vi "InterfaceManagement.vi"() -> ()   [LabVIEW 2019]
uses:
  02 Mode/SerialMode/SerialClass.lvclass
  02 Mode/TCPClientMode/TCPClientClass.lvclass
  02 Mode/TCPServerMode/TCPServerClass.lvclass
  29d042ba-0fcd-46a0-811e-070ad37dbe5e.vi
panel:
  out "新值":string
  in  "更新显示？":bool
  in  "停止":bool
  in  "连接显示":string(tree)
  # "针对客服端/服务端\n不能检测是否可用\n客服端连接服务端的情况，当前无法联动删除"
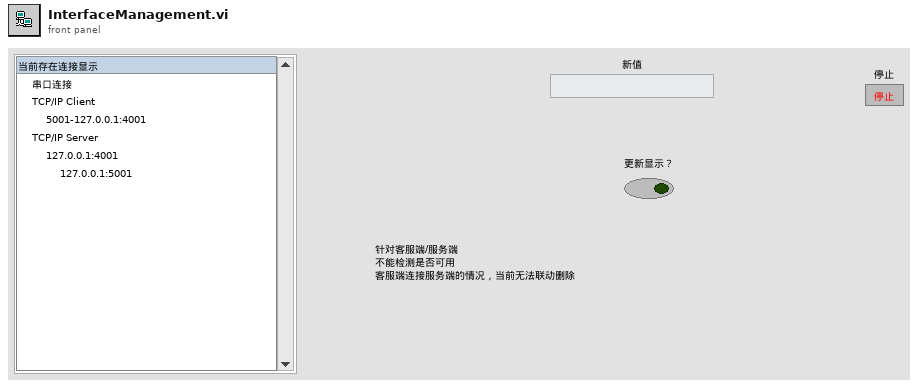
[diagram p1: front panel]
types:
  T1 = typedef "队列枚举1.ctl" = enum16{"接口管理页队列", "服务侦听页队列", "主页队列"}
  T2 = typedef "队列枚举.ctl" = enum16{"ini", "读", "写"}
  T3 = typedef "串口枚举.ctl" = enum16{"ini", "增", "删", "查", "改"}
  T4 = cluster{"串口名":string, "串口类":refnum<class "SerialClass.lvclass">}
  T5 = cluster{"客服名":string, "客服类":refnum<class "TCPClientClass.lvclass">}
  T6 = cluster{"服务名":string, "服务类":refnum<class "TCPServerClass.lvclass">}
  T7 = cluster{"识别名称":string, "记录":cluster{"通讯状态":bool, "记录上限":dbl, "报文记录":string[]}}
  T8 = enum16{"ini", "增", "删", "查", "改-通讯状态", "改-记录上限", "增-报文", "清空报文记录", "清空全部记录"}
  T9 = map{string, refnum<class "TCPClientClass.lvclass">}
  T10 = map{string, refnum<class "TCPServerClass.lvclass">}
  T11 = cluster{"未找到?":bool, "服务类":refnum<class "TCPServerClass.lvclass">}
  T12 = cluster{"字符串":string, "TCPServerClass输出":refnum<class "TCPServerClass.lvclass">}
  T13 = typedef "LVPoint32TypeDef.ctl" = cluster{"Horizontal":i32, "Vertical":i32}
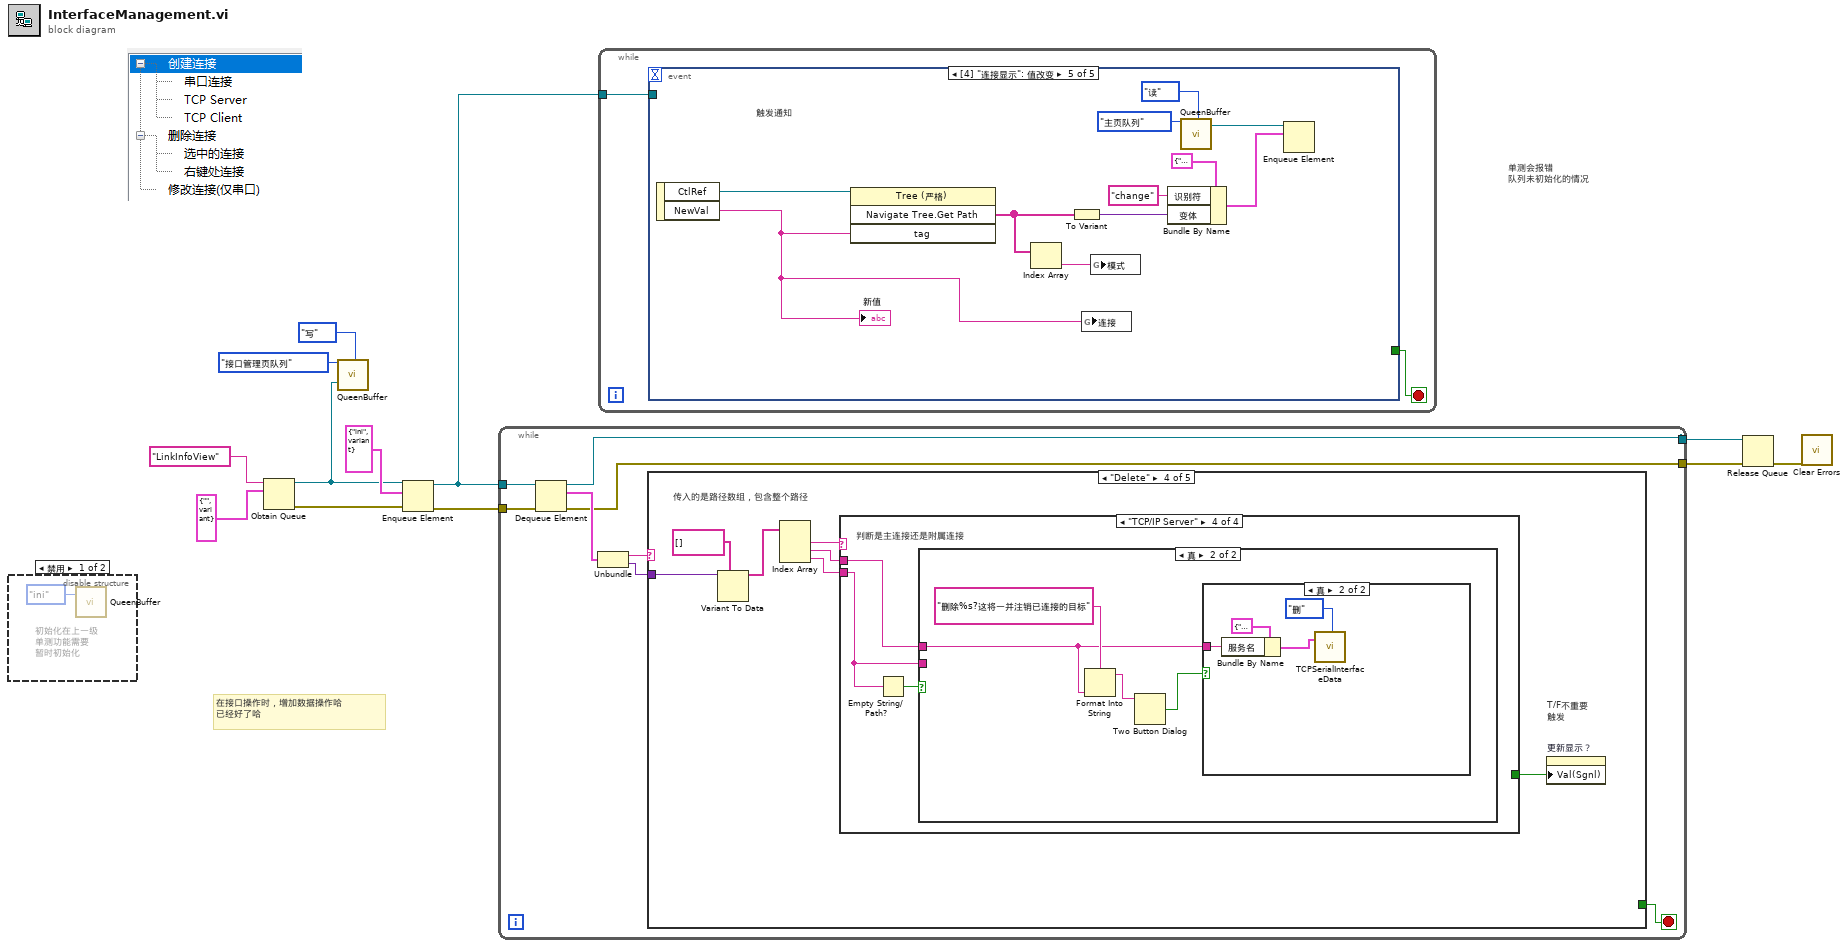
[diagram p0: block diagram]
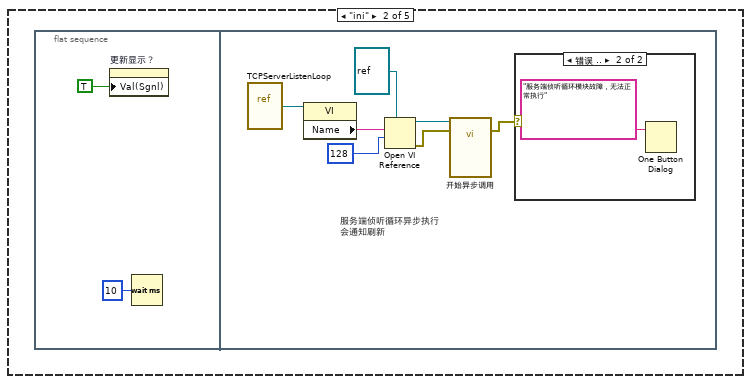
[diagram p4: hidden frame]
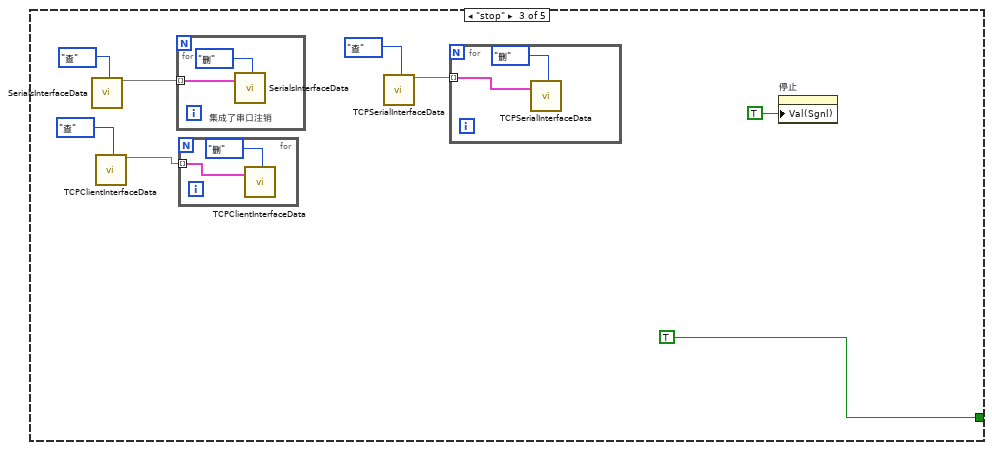
[diagram p6: hidden frame]
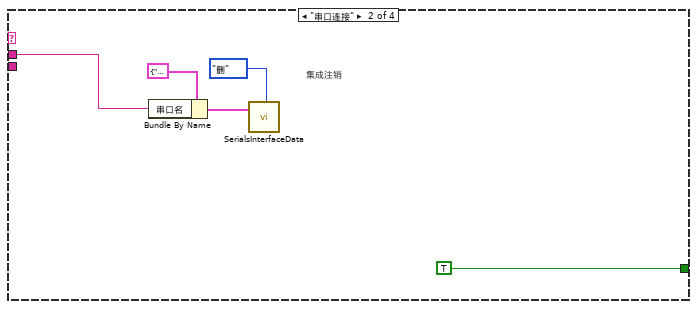
[diagram p8: hidden frame]
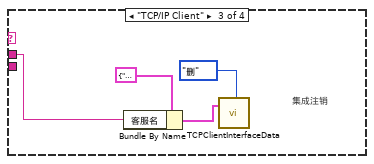
[diagram p9: hidden frame]
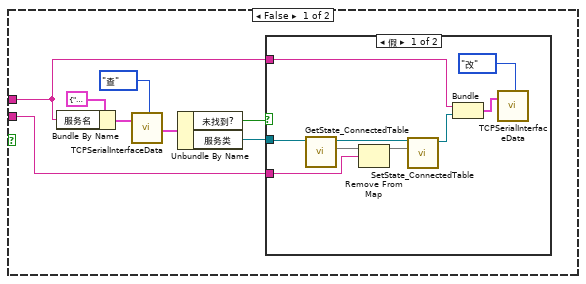
[diagram p10: hidden frame]
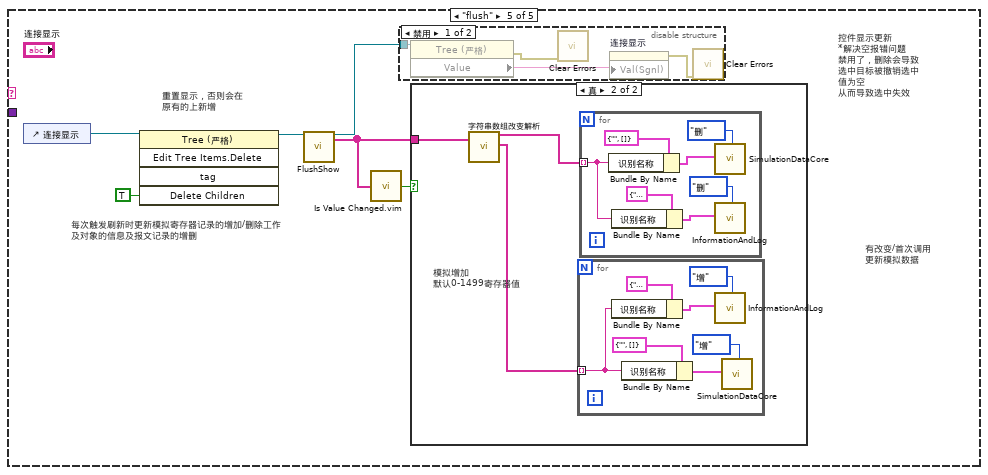
[diagram p13: hidden frame]
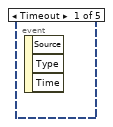
[diagram p16: hidden frame]
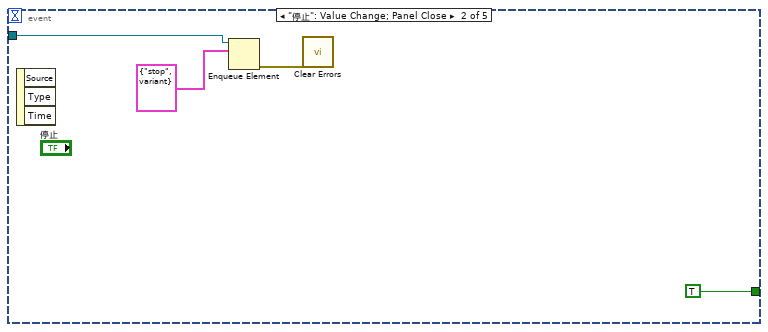
[diagram p17: hidden frame]
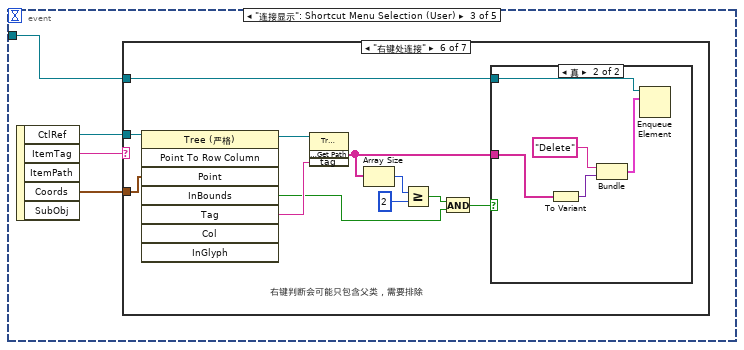
[diagram p18: hidden frame]
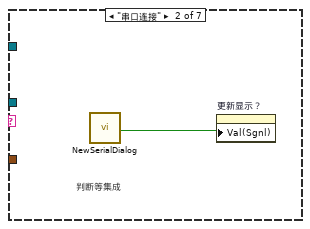
[diagram p20: hidden frame]
diagram:
  # "单测会报错\n队列未初始化的情况"
  # "在接口操作时，增加数据操作哈\n已经好了哈"
  n1 = disable-structure shown="禁用" {
    frame Disabled {
      # "初始化在上一级\n单测功能需要\n暂时初始化"
      n2 = call "QueenBuffer.vi"(1:队列枚举."ini" ("队列枚举")) -> ()  [unwired: 18 in, 1 out]
    }
    frame Enabled {
    }
  }
  n3 = Obtain Queue(name (unnamed)="LinkInfoView" ("名称（未命名）"), element data type=cluster{string, variant} {"", variant}) -> (queue out=w2:refnum<queue>, error out=w11:errorcluster)  [unwired: 3 in, 1 out]
  n4 = call "QueenBuffer.vi"("名称"=队列枚举1."接口管理页队列", "目标队列输入"=w2, "操作"=队列枚举."写") -> ()  [unwired: 16 in, 1 out]
  n5 = Enqueue Element(queue=w2, element=cluster{string, variant} {"ini", variant} ("元素"), error in (no error)=w11) -> (queue out=w10:refnum<queue>, error out=w9:errorcluster)  [unwired: 1 in, 1 out]
  n6 = while {
    tunnel: w10 -> [w21]
    tunnel: w9 -> [w20]
    tunnel: [w16] -> w8
    tunnel: [w15] -> w7
    stop <- w14 stop-if-true
    n7 = Dequeue Element(queue=w21, error in (no error)=w20) -> (queue out=w16:refnum<queue>, element=w19:cluster{string, variant}, error out=w15:errorcluster)  [unwired: 1 in, 1 out]
    n8 = Unbundle(w19) -> (w18:string, w17:variant)
    n9 = case shown="\"Delete\"" w18 {
      tunnel: w17 -> [_ _ _ w52 _]
      tunnel: [_ _ TRUE ("停止") _ _] -> w14
      frame Default {
      }
      frame "ini" {
        n10 = flat-sequence {
          frame #0 {
            n11 = property on="更新显示？" class="Bool (严格)"("Val(Sgnl)"=TRUE ("更新显示？")) -> ()  [unwired: 2 in, 2 out]
            n12 = Wait (ms)(milliseconds to wait=u32 10 ("等待时间（毫秒）")) -> ()  [unwired: 1 out]
          }
          frame #1 {
            # "服务端侦听循环异步执行\n会通知刷新"
            n13 = vi-ref "TCPServerListenLoop.vi"() -> (w30:refnum<vi>)
            n14 = property class="VI"(reference=w30) -> ("Name"=w29:string)  [unwired: 1 in, 2 out]
            n15 = Open VI Reference(type specifier VI Refnum (for type only)=refnum<vi> refnum ("类型说明符VI引用句柄（仅用于类型）"), vi path=w29, options=128 ("选项")) -> (vi reference=w28:refnum<vi>, error out=w27:errorcluster)  [unwired: 3 in]
            n16 = call-by-ref "开始异步调用"(reference=w28, error in=w27) -> (error out=w24:errorcluster)  [unwired: 20 in, 1 out]
            n17 = case shown="错误 .." w24 {
              frame No Error {
              }
              frame Error {
                n18 = One Button Dialog(message="服务端侦听循环模块故障，无法正常执行" ("消息")) -> ()  [unwired: 1 in, 1 out]
              }
            }
          }
        }
      }
      frame "stop" {
        n19 = call "SerialsInterfaceData.vi"("串口枚举"=串口枚举."查") -> ("串口表"=w37:map{string, refnum<class "SerialClass.lvclass">})  [unwired: 17 in, 1 out]
        n20 = call "TCPClientInterfaceData.vi"("客服接口枚举"=enum16{"ini", "增", "删", "查", "改"}."查") -> ("客服表"=w34:T9)  [unwired: 17 in, 1 out]
        n21 = for {
          tunnel: w37 -> [w44] mode=indexing
          # "集成了串口注销"
          n22 = call "SerialsInterfaceData.vi"("信息"=w44, "串口枚举"=串口枚举."删") -> ()  [unwired: 16 in, 2 out]
        }
        n23 = for {
          tunnel: w34 -> [w42] mode=indexing
          n24 = call "TCPClientInterfaceData.vi"("信息"=w42, "客服接口枚举"=enum16{"ini", "增", "删", "查", "改"}."删") -> ()  [unwired: 16 in, 2 out]
        }
        n25 = call "TCPSerialInterfaceData.vi"("客服接口枚举"=enum16{"ini", "增", "删", "查", "改", "腾笼换鸟"}."查") -> ("服务表"=w33:T10)  [unwired: 17 in, 1 out]
        n26 = for {
          tunnel: w33 -> [w40] mode=indexing
          n27 = call "TCPSerialInterfaceData.vi"("信息"=w40, "客服接口枚举"=enum16{"ini", "增", "删", "查", "改", "腾笼换鸟"}."删") -> ()  [unwired: 16 in, 2 out]
        }
        n28 = property on="停止" class="Bool (严格)"("Val(Sgnl)"=TRUE ("值(信号)")) -> ()  [unwired: 2 in, 2 out]
      }
      frame "Delete" {
        # "T/F不重要\n触发"
        # "传入的是路径数组，包含整个路径"
        n29 = Variant To Data(type=string[] [], Variant=w52) -> (data=w50:string[])  [unwired: 1 in, 1 out]
        n30 = Index Array(array=w50) -> (element #1=w49:string, element #2=w48:string, element #3=w47:string)  [unwired: 3 in]
        n31 = case shown="\"TCP/IP Server\"" w49 {
          tunnel: w48 -> [_ w55 w59 w63]
          tunnel: w47 -> [_ _ _ w62]
          tunnel: [_ TRUE _ _] -> w46
          frame Default {
          }
          frame "串口连接" {
            # "集成注销"
            n32 = Bundle By Name(cluster=T4 {"串口名"="", "串口类"=refnum} ("信息"), "串口名"=w55) -> (w54:T4)
            n33 = call "SerialsInterfaceData.vi"("信息"=w54, "串口枚举"=串口枚举."删") -> ()  [unwired: 16 in, 2 out]
          }
          frame "TCP/IP Client" {
            # "集成注销"
            n34 = Bundle By Name(cluster=T5 {"客服名"="", "客服类"=refnum} ("信息"), "客服名"=w59) -> (w58:T5)
            n35 = call "TCPClientInterfaceData.vi"("信息"=w58, "客服接口枚举"=enum16{"ini", "增", "删", "查", "改"}."删") -> ()  [unwired: 16 in, 2 out]
          }
          frame "TCP/IP Server" {
            # "判断是主连接还是附属连接"
            n36 = Empty String/Path?(string/path=w62) -> (empty?=w64:bool)
            n37 = case shown="真" w64 {
              tunnel: w63 -> [w66 w83]
              tunnel: w62 -> [w65 _]
              frame False {
                n38 = Bundle By Name(cluster=T6 {"服务名"="", "服务类"=refnum} ("信息"), "服务名"=w66) -> (w70:T6)
                n39 = call "TCPSerialInterfaceData.vi"("信息"=w70, "客服接口枚举"=enum16{"ini", "增", "删", "查", "改", "腾笼换鸟"}."查") -> ("查找结果"=w69:T11)  [unwired: 16 in, 1 out]
                n40 = Unbundle By Name(w69) -> ("未找到?"=w68:bool, "服务类"=w67:refnum<class "TCPServerClass.lvclass">)
                n41 = case shown="假" w68 {
                  tunnel: w67 -> [w81 _]
                  tunnel: w66 -> [w74 _]
                  tunnel: w65 -> [w78 _]
                  frame False {
                    n42 = call-dynamic "GetState_ConnectedTable.vi"("TCPServerClass输入"=w81) -> ("连接端ID表"=w79:map{string, refnum<k5>}, "TCPServerClass输出"=w80:refnum<class "TCPServerClass.lvclass">)  [unwired: 8 in, 1 out]
                    n43 = Remove From Map(10:w78, 11:w79) -> (3:w77:map{string, refnum<k5>})  [unwired: 2 out]
                    n44 = call-dynamic "SetState_ConnectedTable.vi"("连接端ID表"=w77, "TCPServerClass输入"=w80) -> ("TCPServerClass输出"=w75:refnum<class "TCPServerClass.lvclass">)  [unwired: 8 in, 1 out]
                    n45 = Bundle("字符串"=w74, "TCPServerClass输出"=w75) -> (w73:T12)  [unwired: 1 in]
                    n46 = call "TCPSerialInterfaceData.vi"("信息"=w73, "客服接口枚举"=enum16{"ini", "增", "删", "查", "改", "腾笼换鸟"}."改") -> ()  [unwired: 16 in, 2 out]
                  }
                  frame True {
                  }
                }
              }
              frame True {
                n47 = Format Into String(format string="删除%s?这将一并注销已连接的目标" ("消息"), w83) -> (resulting string=w82:string)  [unwired: 2 in, 1 out]
                n48 = Two Button Dialog(message=w82) -> (T button?=w85:bool)  [unwired: 2 in]
                n49 = case shown="真" w85 {
                  tunnel: w83 -> [_ w87]
                  frame False {
                  }
                  frame True {
                    n50 = Bundle By Name(cluster=T6 {"服务名"="", "服务类"=refnum} ("信息"), "服务名"=w87) -> (w86:T6)
                    n51 = call "TCPSerialInterfaceData.vi"("信息"=w86, "客服接口枚举"=enum16{"ini", "增", "删", "查", "改", "腾笼换鸟"}."删") -> ()  [unwired: 16 in, 2 out]
                  }
                }
              }
            }
          }
        }
        n52 = property on="更新显示？" class="Bool (严格)"("Val(Sgnl)"=w46) -> ()  [unwired: 2 in, 2 out]
      }
      frame "flush" {
        # "每次触发刷新时更新模拟寄存器记录的增加/删除工作\n及对象的信息及报文记录的增删"
        # "有改变/首次调用\n更新模拟数据"
        # "重置显示，否则会在\n原有的上新增"
        # "控件显示更新\n*解决空报错问题\n禁用了，删除会导致\n选中目标被撤销选中\n值为空\n从而导致选中失效"
        n53 = control-ref of="连接显示"() -> (w95:refnum<vi>)
        n54 = invoke on="调用节点" class="Tree (严格)" method="Edit Tree Items.Delete"(reference=w95, "Delete Children"=TRUE ("删除子项？")) -> (reference out=w94:refnum<vi>)  [unwired: 3 in, 4 out]
        n55 = call "FlushShow.vi"("引用输出"=w94) -> ("引用输出"=w90:refnum<vi>, "所有连接名称"=w91:string[])  [unwired: 17 in]
        n56 = call "Is Value Changed.vim"("value"=w91) -> ("changed or first call?"=w92:bool)
        n57 = disable-structure shown="禁用" {
          disable-tunnel: w90 -> [w99 _]
          frame Disabled {
            n58 = property on="属性节点" class="Tree (严格)"(reference=w99) -> (error out=w96:errorcluster, "Value"=w98:string)  [unwired: 1 in, 1 out]
            n59 = call <vilib>:"Clear Errors.vi"("error in (no error)"=w96) -> ()  [unwired: 5 in, 2 out]
            n60 = property on="连接显示" class="Tree (严格)"("Val(Sgnl)"=w98) -> (error out=w97:errorcluster)  [unwired: 2 in, 1 out]
            n61 = call <vilib>:"Clear Errors.vi"("error in (no error)"=w97) -> ()  [unwired: 5 in, 2 out]
          }
          frame Enabled {
          }
        }
        n62 = case shown="真" w92 {
          tunnel: w91 -> [_ w102]
          frame False {
          }
          frame True {
            # "模拟增加\n默认0-1499寄存器值"
            n63 = call "字符串数组改变解析.vi"("字符串数组"=w102) -> ("删除"=w100:string[], "新增"=w101:string[])  [unwired: 17 in]
            n64 = for {
              tunnel: w101 -> [w103] mode=indexing
              n65 = Bundle By Name(cluster=T7 {"识别名称"="", "记录"={"通讯状态"=FALSE, "记录上限"=0.0, "报文记录"=[]}} ("配置信息"), "识别名称"=w103) -> (w106:T7)
              n66 = Bundle By Name(cluster=cluster{"识别名称":string, "模拟寄存器":u16[]} {"识别名称"="", "模拟寄存器"=[]} ("配置信息"), "识别名称"=w103) -> (w107:cluster{"识别名称":string, "模拟寄存器":u16[]})
              n67 = call "InformationAndLog.vi"("配置信息"=w106, "模拟数据枚举"=T8."增") -> ()  [unwired: 16 in, 2 out]
              n68 = call "SimulationDataCore.vi"("配置信息"=w107, "模拟数据枚举"=enum16{"ini", "增", "删", "查", "改-全", "改-部分"}."增") -> ()  [unwired: 16 in, 2 out]
            }
            n69 = for {
              tunnel: w100 -> [w110] mode=indexing
              n70 = Bundle By Name(cluster=cluster{"识别名称":string, "模拟寄存器":u16[]} {"识别名称"="", "模拟寄存器"=[]} ("配置信息"), "识别名称"=w110) -> (w114:cluster{"识别名称":string, "模拟寄存器":u16[]})
              n71 = Bundle By Name(cluster=T7 {"识别名称"="", "记录"={"通讯状态"=FALSE, "记录上限"=0.0, "报文记录"=[]}} ("配置信息"), "识别名称"=w110) -> (w111:T7)
              n72 = call "SimulationDataCore.vi"("配置信息"=w114, "模拟数据枚举"=enum16{"ini", "增", "删", "查", "改-全", "改-部分"}."删") -> ()  [unwired: 16 in, 2 out]
              n73 = call "InformationAndLog.vi"("配置信息"=w111, "模拟数据枚举"=T8."删") -> ()  [unwired: 16 in, 2 out]
            }
          }
        }
      }
    }
  }
  n74 = while {
    tunnel: w10 -> [w117]
    stop <- w118 stop-if-true
    n75 = event shown="[4] \"连接显示\": 值改变" {
      selector: _ -> [_ _ _ _ _]
      dyn-events: _ -> [_ _ _ _ _]
      timeout: _ -> [_ _ _ _ _]
      tunnel: [_ TRUE ("停止") _ _ _] -> w118
      tunnel: w117 -> [_ w121 w125 w160 _]
      event Timeout {
        n76 = event-data() -> ()  [unwired: 1 in, 3 out]
      }
      event "停止": Value Change; Panel Close {
        n77 = event-data() -> ()  [unwired: 1 in, 3 out]
        n78 = Enqueue Element(queue=w121, element=cluster{string, variant} {"stop", variant} ("元素")) -> (error out=w119:errorcluster)  [unwired: 2 in, 2 out]
        n79 = call <vilib>:"Clear Errors.vi"("error in (no error)"=w119) -> ()  [unwired: 5 in, 2 out]
      }
      event "连接显示": Shortcut Menu Selection (User) {
        n80 = event-data() -> ("CtlRef"=w124:refnum<vi>, "ItemTag"=w126:string, "Coords"=w123:T13)  [unwired: 1 in, 2 out]
        n81 = case shown="\"右键处连接\"" w126 {
          tunnel: w125 -> [_ _ _ _ w135 w152 _]
          tunnel: w124 -> [_ _ _ _ w134 w151 _]
          tunnel: w123 -> [_ _ _ _ _ w150 _]
          frame Default {
          }
          frame "串口连接" {
            # "判断等集成"
            n82 = call "NewSerialDialog.vi"() -> ("执行完毕"=w127:bool)  [unwired: 19 in]
            n83 = property on="更新显示？" class="Bool (严格)"("Val(Sgnl)"=w127) -> ()  [unwired: 2 in, 2 out]
          }
          frame "TCP Server" {
            # "持续循环侦听功能分离\n独立执行侦听"
            n84 = call "NewTCPServerDialog.vi"() -> ("执行完成"=w128:bool)  [unwired: 19 in]
            n85 = property on="更新显示？" class="Bool (严格)"("Val(Sgnl)"=w128) -> ()  [unwired: 2 in, 2 out]
          }
          frame "TCP Client" {
            n86 = call "NewTCPClientDialog.vi"() -> ("执行结束"=w129:bool)  [unwired: 19 in]
            n87 = property on="更新显示？" class="Bool (严格)"("Val(Sgnl)"=w129) -> ()  [unwired: 2 in, 2 out]
          }
          frame "选中的连接" {
            # "设置了父类不可选中的"
            n88 = property class="Tree (严格)"(reference=w134) -> (reference out=w132:refnum<vi>, "Value"=w133:string)  [unwired: 1 in, 1 out]
            n89 = invoke class="Tree (严格)" method="Navigate Tree.Get Path"(reference=w132, "tag"=w133) -> ("Navigate Tree:Get Path"=w130:string[])  [unwired: 2 in, 3 out]
            n90 = Empty Array?(array=w130) -> (empty?=w131:bool)
            n91 = case shown="假" w131 {
              tunnel: w135 -> [w140 _]
              tunnel: w130 -> [w136 _]
              frame False {
                n92 = To Variant(anything=w136) -> (Variant=w139:variant)
                n93 = Bundle("Delete", "Variant"=w139) -> (w138:cluster{string, "Variant":variant})  [unwired: 1 in]
                n94 = Enqueue Element(queue=w140, element=w138) -> ()  [unwired: 2 in, 3 out]
              }
              frame True {
                n95 = One Button Dialog(message="啥都没有选啊" ("消息")) -> ()  [unwired: 1 in, 1 out]
              }
            }
          }
          frame "右键处连接" {
            # "右键判断会可能只包含父类，需要排除"
            n96 = invoke class="Tree (严格)" method="Point To Row Column"(reference=w151, "Point"=w150) -> (reference out=w149:refnum<vi>, "InBounds"=w143:bool, "Tag"=w148:string)  [unwired: 6 in, 5 out]
            n97 = invoke class="Tree (严格)" method="Navigate Tree.Get Path"(reference=w149, "tag"=w148) -> ("Navigate Tree:Get Path"=w147:string[])  [unwired: 2 in, 3 out]
            n98 = Array Size(array=w147) -> (size(s)=w146:i32)
            n99 = Greater Or Equal?(x=w146, y=2) -> (x >= y?=w144:bool)
            n100 = And(x=w144, y=w143) -> (x .and. y?=w142:bool)
            n101 = case shown="真" w142 {
              tunnel: w152 -> [_ w156]
              tunnel: w147 -> [_ w154]
              frame False {
                n102 = One Button Dialog(message="选择错误，请选择连接" ("消息")) -> ()  [unwired: 1 in, 1 out]
              }
              frame True {
                n103 = To Variant(anything=w154) -> (Variant=w158:variant)
                n104 = Bundle("Delete", "Variant"=w158) -> (w157:cluster{string, "Variant":variant})  [unwired: 1 in]
                n105 = Enqueue Element(queue=w156, element=w157) -> ()  [unwired: 2 in, 3 out]
              }
            }
          }
          frame "修改连接" {
            # "已删除"
          }
        }
      }
      event "更新显示？": Value Change {
        n106 = event-data() -> ()  [unwired: 1 in, 6 out]
        n107 = Enqueue Element(queue=w160, element=cluster{string, variant} {"flush", variant} ("元素")) -> ()  [unwired: 2 in, 3 out]
      }
      event "连接显示": Value Change {
        # "触发通知"
        n108 = event-data() -> ("CtlRef"=w167:refnum<vi>, "NewVal"=w163:string)  [unwired: 1 in]
        "新值" <- w163
        n109 = invoke class="Tree (严格)" method="Navigate Tree.Get Path"(reference=w167, "tag"=w163) -> ("Navigate Tree:Get Path"=w162:string[])  [unwired: 2 in, 3 out]
        n110 = Index Array(array=w162) -> (element=w161:string)  [unwired: 1 in]
        n111 = To Variant(anything=w162) -> (Variant=w164:variant)
        n112 = global write "全局-配置识别.vi" "连接"(w163) -> ()
        n113 = global write "全局-配置识别.vi" "模式"(w161) -> ()
        n114 = Bundle By Name(cluster=cluster{"识别符":string, "变体":variant} {"识别符"="", "变体"=variant} ("元素"), "识别符"="change", "变体"=w164) -> (w168:cluster{"识别符":string, "变体":variant})
        n115 = call "QueenBuffer.vi"("名称"=enum16{"接口管理页队列", "服务侦听页队列", "主页队列"}."主页队列", "操作"=队列枚举."读") -> ("目标队列"=w171:refnum<queue>)  [unwired: 17 in]
        n116 = Enqueue Element(queue=w171, element=w168) -> ()  [unwired: 2 in, 3 out]
      }
    }
  }
  n117 = Release Queue(queue=w8, error in (no error)=w7) -> (error out=w6:errorcluster)  [unwired: 1 in, 2 out]
  n118 = call <vilib>:"Clear Errors.vi"("error in (no error)"=w6) -> ()  [unwired: 5 in, 2 out]
